vi "指定时刻（时分秒）闹钟.vi"(8 "Error In":errorcluster caption="错误输入", 9 "模式":enum16{"秒", "分", "时"}(ring), 10 "偏移量":i32) -> (0 "Error Out":errorcluster caption="错误输出", 1 "时刻":i32, 3 "时间到":bool)   [LabVIEW 2012]
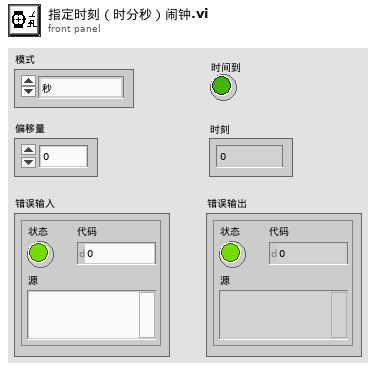
[diagram p1: front panel]
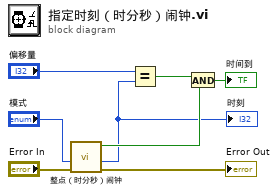
[diagram p0: block diagram]
diagram:
  n1 = call "整点（时分秒）闹钟.vi"("Error In"="Error In", "模式"="模式") -> ("Error Out"=→"Error Out":errorcluster, "时刻"=w1:i32, "时间到"=w4:bool)  [unwired: 7 in]
  "时刻" <- w1
  n2 = Equal?(x="偏移量", y=w1) -> (x = y?=w3:bool)
  n3 = And(x=w3, y=w4) -> (x .and. y?=→"时间到":bool)
